vi "Time Stamp-old.vi"(2 "Point #":i32) -> (0 "Stop":bool, 1 "Time Stamp (Sec)":dbl[](array[numeric]) format="%.2f")   [LabVIEW 2025]
doc: "Returns time in seconds since point number zero.\nScott Hannahs, FBNML, May 1993\nAuthor: Scott Hannahs <sth@magnet.fsu.edu>\n\nThis software is licensed for use under the “MIT License\"\nCopyright (c) 2025 Scott Hannahs, sth@sth@magnet.sthnet.net\n\nPermission is hereby granted, free of charge, to any person obtaining a copy of this software and associated documentation files (the \"Software\"), to deal in the Software without restriction, including without limitation the rights to use, copy, modify, merge, publish, distribute, sublicense, and/or sell copies of the Software, and to permit persons to whom the Software is furnished to do so, subject to the following conditions: The above copyright notice and this permission notice shall be included in all copies or substantial portions of the Software.\n\nTHE SOFTWARE IS PROVIDED \"AS IS\", WITHOUT WARRANTY OF ANY KIND, EXPRESS OR IMPLIED, INCLUDING BUT NOT LIMITED TO THE WARRANTIES OF MERCHANTABILITY, FITNESS FOR A PARTICULAR PURPOSE AND NONINFRINGEMENT. IN NO EVENT SHALL THE AUTHORS OR COPYRIGHT HOLDERS BE LIABLE FOR ANY CLAIM, DAMAGES OR OTHER LIABILITY, WHETHER IN AN ACTION OF CONTRACT, TORT OR OTHERWISE, ARISING FROM, OUT OF OR IN CONNECTION WITH THE SOFTWARE OR THE USE OR OTHER DEALINGS IN THE SOFTWARE."
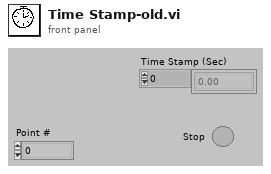
[diagram p1: front panel]
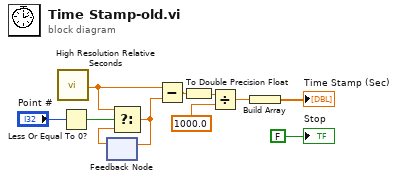
[diagram p0: block diagram]
diagram:
  n1 = call <vilib>:"High Resolution Relative Seconds.vi"() -> ("relative seconds"=w1:dbl)
  n2 = Less Or Equal To 0?(x="Point #") -> (x <= 0?=w7:bool)
  n3 = feedback #1() -> (w6:dbl)  [unwired: 1 in]
  n4 = Select(t=w1, s=w7, f=w6) -> (s? t:f=w5:dbl)
  n5 = feedback-in #1(w5) -> ()
  n6 = Subtract(x=w1, y=w5) -> (x-y=w3:dbl)
  n7 = To Double Precision Float(number=w3) -> (double precision float=w2:dbl)
  n8 = Divide(x=w2, y=1000.0) -> (x/y=w11:dbl)
  n9 = Build Array(w11) -> (→"Time Stamp (Sec)":dbl[])
  "Stop" <- FALSE
